vi "Zeiss Teleoperation.vi"(8 "error in":errorcluster) -> (0 "error out":errorcluster)   [LabVIEW 2016]
uses:
  <vilib>/Platform/TimedLoop/XDataNode/timing_clust.ctl
  <vilib>/Platform/TimedLoop/XDataNode/nitl_modes.ctl
  <vilib>/Platform/TimedLoop/XDataNode/wakeup.ctl
  Subsystems/Global Variables.vi
  <vilib>/platform/TimedLoop/XDataNode/XDataNode.xnode
  <vilib>/Platform/TimedLoop/XDataNode/XDNodeRunTimeDep.lvlib
panel:
  out "vac cmd":dbl
  out "Hydration On/Off":bool
  out "q5 cmd":dbl
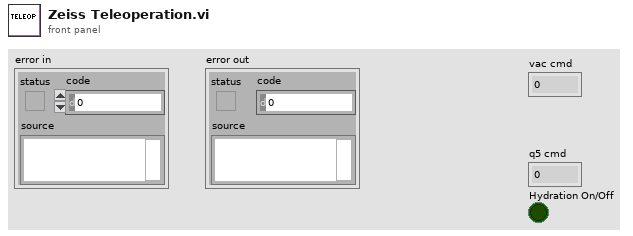
[diagram p1: front panel]
types:
  T1 = typedef "XDNodeRunTimeDep.lvlib/timing_clust.ctl" = cluster{"Expected End [f-1]":u64, "Actual End [f-1]":u64, "Finished Late? [f-1]":bool, "Expected End [i-1]":u64, "Actual End [i-1]":u64, "Finished Late? [i-1]":bool, "Expected Start [i]":u64, "Actual Start [i]":u64, "Expected Start [f]":u64, "Actual Start [f]":u64, "Source Name":string, "Structure Name":string, "Period":i64, "Deadline":i64, "Offset":i64, "Start":i64, "Priority":i32, "Timeout":i32, "Mode":T2, "Wakeup Reason":T3, "Error":errorcluster, "Source Type":string, "Secondary Source Type":string, "Global End Time":u64, "Global Start Time":u64, "Frame Duration":u64, "Iteration Duration":u64, "Assigned CPU":i32, "I/O Scan Engine Mode":u32}
  T2 = typedef "XDNodeRunTimeDep.lvlib/nitl_modes.ctl" = enum32{"No Change", "Process missed periods, maintain original phase", "Discard missed periods, maintain original phase", "Process missed periods, ignore original phase", "Discard missed periods, ignore original phase"}
  T3 = typedef "XDNodeRunTimeDep.lvlib/wakeup.ctl" = enum32{"Normal", "Aborted", "Asynchronous wakeup", "Timing source error", "Timed loop error", "Timeout"}
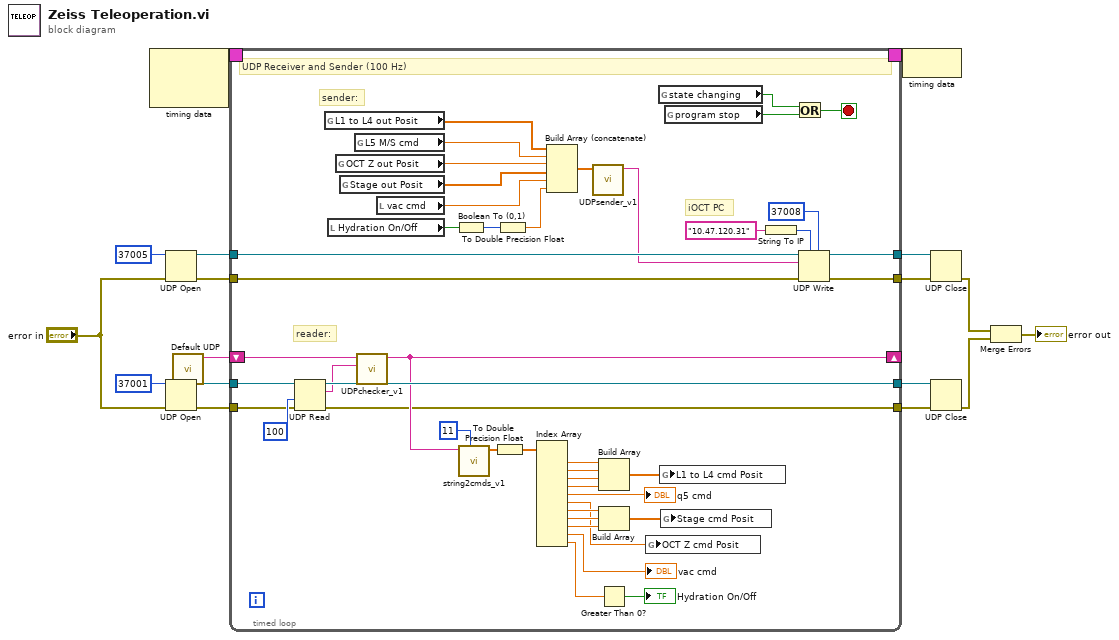
[diagram p0: block diagram]
diagram:
  n1 = node-c288() -> (w17:T1)  [unwired: 2 in]
  n2 = UDP Open(8:"error in", 11:u16 37005 ("port")) -> (port=w11:refnum<k16>, 0:w10:errorcluster)  [unwired: 3 in, 1 out]
  n3 = UDP Open(8:"error in", 11:u16 37001 ("port")) -> (port=w14:refnum<k16>, 0:w7:errorcluster)  [unwired: 3 in, 1 out]
  n4 = call "Default UDP.vi"() -> ("String"=w5:string)  [unwired: 11 in]
  n5 = timed-loop {
    timing: w17 -> [_]
    timing-out: [_] -> w16
    tunnel: w14 -> [w61]
    tunnel: [w60] -> w13
    shift-right: [w44] -> _
    shift-left: w5 -> [w45]
    tunnel: w11 -> [w42]
    tunnel: w10 -> [w41]
    tunnel: [w37] -> w8
    tunnel: [w36] -> w9
    tunnel: w7 -> [w35]
    tunnel: [w34] -> w6
    stop <- w18 stop-if-true
    # "sender:"
    # "reader:"
    # "iOCT PC"
    # "UDP Receiver and Sender (100 Hz)"
    n6 = UDP Read(connection ID=w61, timeout ms (25000)=100, 8:w35) -> (data out=w43:string, error out=w34:errorcluster, 3:w60:refnum<k16>)  [unwired: 1 in, 2 out]
    n7 = global read "Global Variables.vi" "L1 to L4 out Posit"() -> (w27:dbl[])
    n8 = local read "Hydration On/Off"() -> (w30:bool)
    n9 = global read "Global Variables.vi" "OCT Z out Posit"() -> (w25:dbl)
    n10 = global read "Global Variables.vi" "Stage out Posit"() -> (w24:dbl[])
    n11 = global read "Global Variables.vi" "L5 M/S cmd"() -> (w26:dbl)
    n12 = call "UDPchecker_v1.vi"("new string"=w43, "old string"=w45) -> ("output string"=w44:string)  [unwired: 9 in]
    n13 = local read "vac cmd"() -> (w31:dbl)
    n14 = Boolean To (0,1)(Boolean=w30) -> (0, 1=w29:i16)
    n15 = call "string2cmds_v1.vi"("numCmds"=11, "input string"=w44) -> ("output cmds"=w50:sgl[])  [unwired: 9 in]
    n16 = To Double Precision Float(number=w50) -> (double precision float=w49:dbl[])
    n17 = To Double Precision Float(number=w29) -> (double precision float=w28:dbl)
    n18 = Index Array(array=w49) -> (element #1=w58:dbl, element #2=w57:dbl, element #3=w56:dbl, element #4=w55:dbl, element #5=→"q5 cmd":dbl, element #6=w21:dbl, element #7=w53:dbl, element #8=w52:dbl, element #9=w51:dbl, element #10=→"vac cmd":dbl, element #11=w47:dbl)  [unwired: 11 in]
    n19 = Build Array (concatenate)(w27, w26, w25, w24, w31, w28) -> (w32:dbl[])
    n20 = call "UDPsender_v1.vi"("nums2send"=w32) -> ("string2send"=w33:string)  [unwired: 10 in]
    n21 = Build Array(w58, w57, w56, w55) -> (w23:dbl[])
    n22 = Build Array(w53, w52, w51) -> (w22:dbl[])
    n23 = Greater Than 0?(x=w47) -> (x > 0?=→"Hydration On/Off":bool)
    n24 = global write "Global Variables.vi" "OCT Z cmd Posit"(w21) -> ()
    n25 = global read "Global Variables.vi" "state changing"() -> (w20:bool)
    n26 = global write "Global Variables.vi" "L1 to L4 cmd Posit"(w23) -> ()
    n27 = global write "Global Variables.vi" "Stage cmd Posit"(w22) -> ()
    n28 = global read "Global Variables.vi" "program stop"() -> (w19:bool)
    n29 = String To IP(1:"10.47.120.31" ("name")) -> (0:w39:u32)
    n30 = Or(x=w20, y=w19) -> (x .or. y?=w18:bool)
    n31 = UDP Write(address=w39, port or service name=u16 37008, connection ID=w42, data in=w33, 8:w41) -> (error out=w36:errorcluster, 3:w37:refnum<k16>)  [unwired: 1 in]
  }
  n32 = node-c288(w16) -> ()
  n33 = UDP Close(connection ID=w8, 8:w9) -> (error out=w3:errorcluster)  [unwired: 1 out]
  n34 = UDP Close(connection ID=w13, 8:w6) -> (error out=w2:errorcluster)  [unwired: 1 out]
  n35 = Merge Errors(w3, w2) -> (→"error out":errorcluster)
